vi "VI Tree.vi"   [LabVIEW 2020, in "Keithley 648X Series.lvlib"]
doc: "This is the instrument driver for the Keithley 648X Series of picoammeters. \nVI Tree displays all the user-callable VIs of the instrument driver in an organized table.\n<b>Note: </b>Model 6482 is not supported"
uses:
  <instrlib>/Keithley 648X Series/Keithley 648X Series.lvlib
panel:
  # "(c) 2017 National Instruments.  ALL RIGHTS RESERVED."
  # "SEE DIAGRAM\nFOR VI TREE."
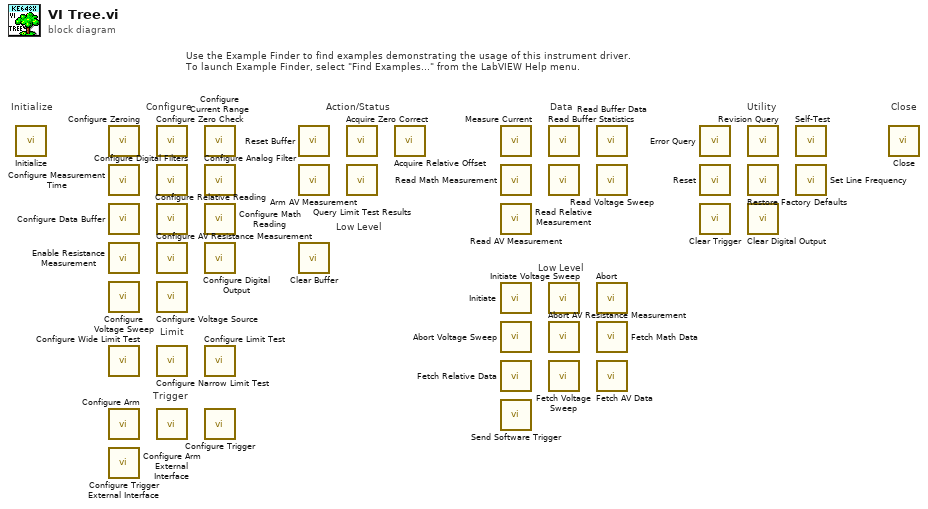
[diagram p0: block diagram]
diagram:
  # "Low Level"
  # "Trigger"
  # "Limit"
  # "Action/Status"
  # "Low Level"
  # "Use the Example Finder to find examples demonstrating the usage of this instrument driver.\nTo launch Example Finder, select \"Find Examples...\" from the LabVIEW Help menu."
  # "Configure"
  # "Utility"
  # "Data"
  # "Close"
  # "Initialize"
  n1 = call <instrlib>:"Initialize.vi"() -> ()  [unwired: 10 in, 2 out]
  n2 = call <instrlib>:"Configure Zeroing.vi"() -> ()  [unwired: 14 in, 2 out]
  n3 = call <instrlib>:"Configure Measurement Time.vi"() -> ()  [unwired: 14 in, 2 out]
  n4 = call <instrlib>:"Configure Data Buffer.vi"() -> ()  [unwired: 14 in, 2 out]
  n5 = call <instrlib>:"Enable Resistance Measurement.vi"() -> ()  [unwired: 14 in, 2 out]
  n6 = call <instrlib>:"Configure Voltage Sweep.vi"() -> ()  [unwired: 14 in, 2 out]
  n7 = call <instrlib>:"Configure Wide Limit Test.vi"() -> ()  [unwired: 14 in, 2 out]
  n8 = call <instrlib>:"Configure Arm.vi"() -> ()  [unwired: 14 in, 2 out]
  n9 = call <instrlib>:"Configure Trigger External Interface.vi"() -> ()  [unwired: 14 in, 2 out]
  n10 = call <instrlib>:"Configure Zero Check.vi"() -> ()  [unwired: 14 in, 2 out]
  n11 = call <instrlib>:"Configure Digital Filters.vi"() -> ()  [unwired: 14 in, 2 out]
  n12 = call <instrlib>:"Configure Relative Reading.vi"() -> ()  [unwired: 14 in, 2 out]
  n13 = call <instrlib>:"Configure AV Resistance Measurement.vi"() -> ()  [unwired: 14 in, 2 out]
  n14 = call <instrlib>:"Configure Voltage Source.vi"() -> ()  [unwired: 14 in, 2 out]
  n15 = call <instrlib>:"Configure Narrow Limit Test.vi"() -> ()  [unwired: 14 in, 2 out]
  n16 = call <instrlib>:"Configure Arm External Interface.vi"() -> ()  [unwired: 14 in, 2 out]
  n17 = call <instrlib>:"Configure Current Range.vi"() -> ()  [unwired: 14 in, 2 out]
  n18 = call <instrlib>:"Configure Analog Filter.vi"() -> ()  [unwired: 14 in, 2 out]
  n19 = call <instrlib>:"Configure Math Reading.vi"() -> ()  [unwired: 14 in, 2 out]
  n20 = call <instrlib>:"Configure Digital Output.vi"() -> ()  [unwired: 14 in, 2 out]
  n21 = call <instrlib>:"Configure Limit Test.vi"() -> ()  [unwired: 14 in, 2 out]
  n22 = call <instrlib>:"Configure Trigger.vi"() -> ()  [unwired: 14 in, 2 out]
  n23 = call <instrlib>:"Reset Buffer.vi"() -> ()  [unwired: 14 in, 2 out]
  n24 = call <instrlib>:"Arm AV Measurement.vi"() -> ()  [unwired: 14 in, 2 out]
  n25 = call <instrlib>:"Clear Buffer.vi"() -> ()  [unwired: 14 in, 2 out]
  n26 = call <instrlib>:"Acquire Zero Correct.vi"() -> ()  [unwired: 14 in, 2 out]
  n27 = call <instrlib>:"Query Limit Test Results.vi"() -> ()  [unwired: 12 in, 4 out]
  n28 = call <instrlib>:"Acquire Relative Offset.vi"() -> ()  [unwired: 14 in, 2 out]
  n29 = call <instrlib>:"Measure Current.vi"() -> ()  [unwired: 13 in, 3 out]
  n30 = call <instrlib>:"Read Math Measurement.vi"() -> ()  [unwired: 13 in, 3 out]
  n31 = call <instrlib>:"Read AV Measurement.vi"() -> ()  [unwired: 13 in, 3 out]
  n32 = call <instrlib>:"Initiate.vi"() -> ()  [unwired: 14 in, 2 out]
  n33 = call <instrlib>:"Abort Voltage Sweep.vi"() -> ()  [unwired: 14 in, 2 out]
  n34 = call <instrlib>:"Fetch Relative Data.vi"() -> ()  [unwired: 13 in, 3 out]
  n35 = call <instrlib>:"Send Software Trigger.vi"() -> ()  [unwired: 14 in, 2 out]
  n36 = call <instrlib>:"Read Buffer Statistics.vi"() -> ()  [unwired: 9 in, 7 out]
  n37 = call <instrlib>:"Read Relative Measurement.vi"() -> ()  [unwired: 13 in, 3 out]
  n38 = call <instrlib>:"Initiate Voltage Sweep.vi"() -> ()  [unwired: 10 in, 2 out]
  n39 = call <instrlib>:"Abort AV Resistance Measurement.vi"() -> ()  [unwired: 14 in, 2 out]
  n40 = call <instrlib>:"Fetch Voltage Sweep.vi"() -> ()  [unwired: 13 in, 3 out]
  n41 = call <instrlib>:"Read Buffer Data.vi"() -> ()  [unwired: 13 in, 3 out]
  n42 = call <instrlib>:"Read Voltage Sweep.vi"() -> ()  [unwired: 13 in, 3 out]
  n43 = call <instrlib>:"Abort.vi"() -> ()  [unwired: 14 in, 2 out]
  n44 = call <instrlib>:"Fetch Math Data.vi"() -> ()  [unwired: 13 in, 3 out]
  n45 = call <instrlib>:"Fetch AV Data.vi"() -> ()  [unwired: 13 in, 3 out]
  n46 = call <instrlib>:"Error Query.vi"() -> ()  [unwired: 8 in, 4 out]
  n47 = call <instrlib>:"Reset.vi"() -> ()  [unwired: 14 in, 2 out]
  n48 = call <instrlib>:"Clear Trigger.vi"() -> ()  [unwired: 14 in, 2 out]
  n49 = call <instrlib>:"Revision Query.vi"() -> ()  [unwired: 8 in, 4 out]
  n50 = call <instrlib>:"Restore Factory Defaults.vi"() -> ()  [unwired: 14 in, 2 out]
  n51 = call <instrlib>:"Clear Digital Output.vi"() -> ()  [unwired: 14 in, 2 out]
  n52 = call <instrlib>:"Self-Test.vi"() -> ()  [unwired: 8 in, 4 out]
  n53 = call <instrlib>:"Set Line Frequency.vi"() -> ()  [unwired: 14 in, 2 out]
  n54 = call <instrlib>:"Close.vi"() -> ()  [unwired: 11 in, 1 out]
